vi "Evaluate Alarms.vi"(0 "In Test":bool, 1 "Controller":T2, 2 "Alarm Config":T3, 3 "Data":dbl[](array[numeric]), 4 "Pumps Present":u32, 5 "Trip Counter":i32[](array[numeric]), 6 "Previous Times":u32[](array[numeric]), 7 "Manual CMDs":dbl[](array[numeric]), 9 "Prev ON Times":u32[](array[numeric])) -> (20 "Trip Counter OUT":i32[](array[numeric]), 21 "Previous Times OUT":u32[](array[numeric]), 22 "Alarm Tripped":bool, 23 "Alarm Message":string, 24 "Prev ON Times OUT":u32[](array[numeric]))   [LabVIEW 2019]
uses:
  Controls/Alarm Config.ctl
  Controls/Alarm Definition.ctl
  Controls/Alarm Profile Config.ctl
  Type Defs/Controller Names.ctl
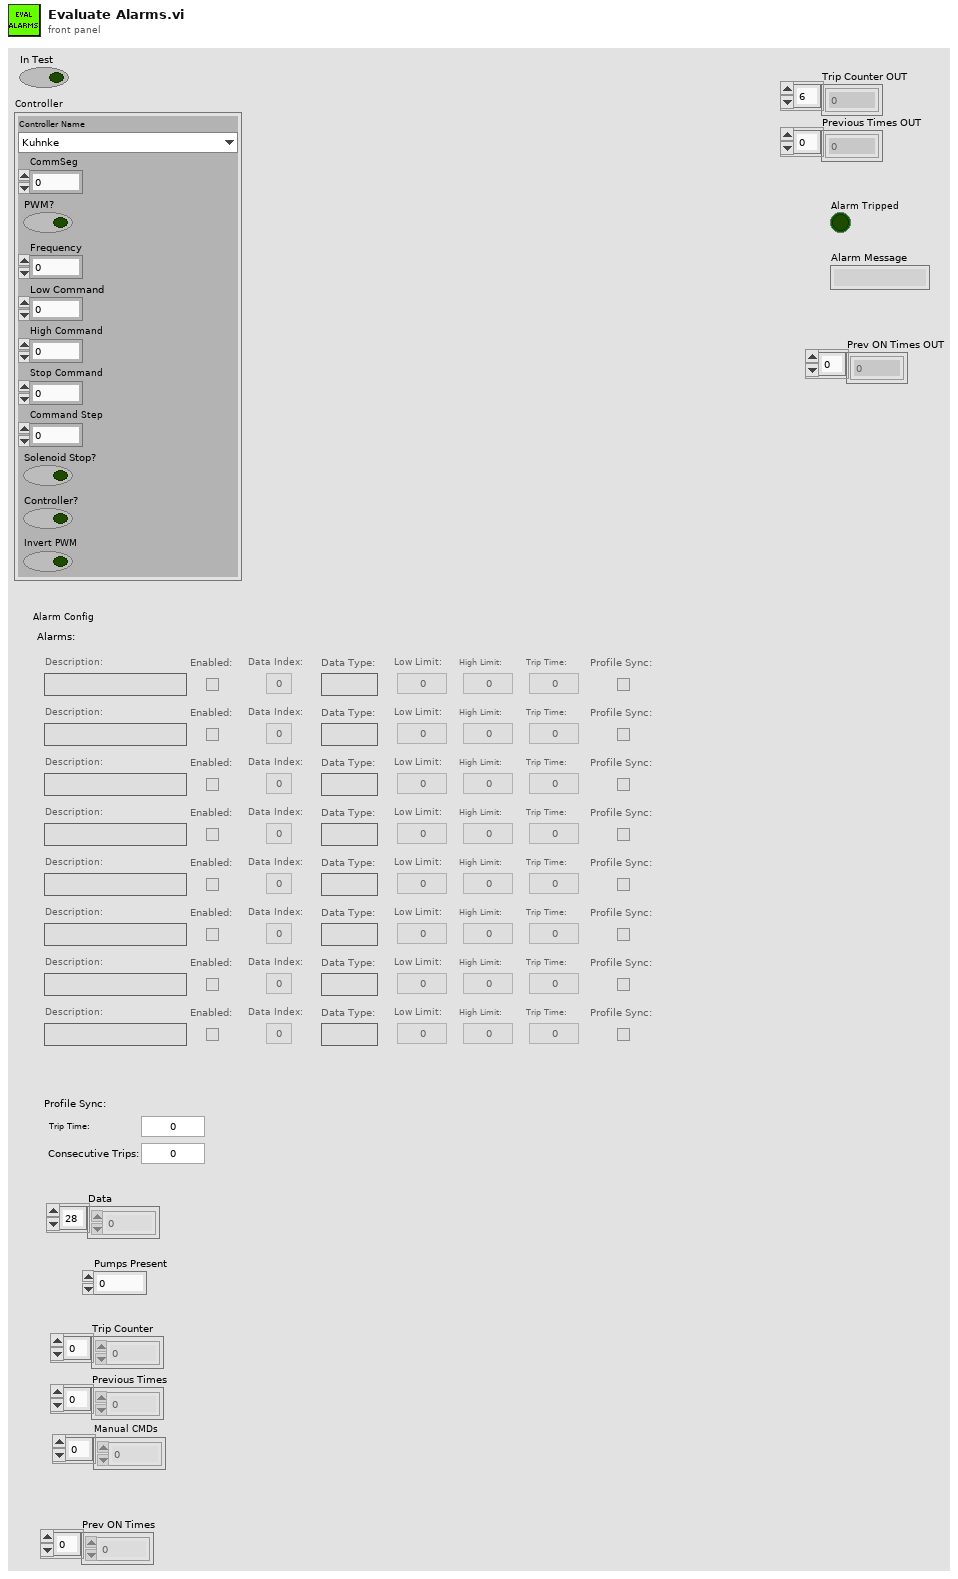
[diagram p1: front panel]
types:
  T1 = typedef "Controller Names.ctl" = enum16{"Kuhnke", "Conti", "Hella BLDC OL PWM", "Hella BLDC Turbine OL PWM", "Helbako", "TI PWM", "PSA", "Hella DC Gas", "Hella DC Diesel", "8 Comm", "10 Comm", "8 Comm Hella", "10 Comm Hella", "8 Comm Omron", "10 Comm Omron", "8 Comm Nissan", "10 Comm Nissan"}
  T2 = cluster{"Controller Name":T1, "CommSeg":i32, "PWM?":bool, "Frequency":i32, "Low Command":dbl, "High Command":dbl, "Stop Command":dbl, "Command Step":dbl, "Solenoid Stop?":bool, "Controller?":bool, "Invert PWM":bool}
  T3 = typedef "Alarm Config.ctl" = cluster{"Alarms:":T4[], "Profile Sync:":T5}
  T4 = typedef "Alarm Definition.ctl" = cluster{"Description:":string, "Enabled:":bool, "Data Index:":i32, "Data Type:":string, "Low Limit:":dbl, "High Limit:":dbl, "Trip Time:":u32, "Profile Sync:":bool}
  T5 = typedef "Alarm Profile Config.ctl" = cluster{"Trip Time:":u32, "Consecutive Trips:":i32}
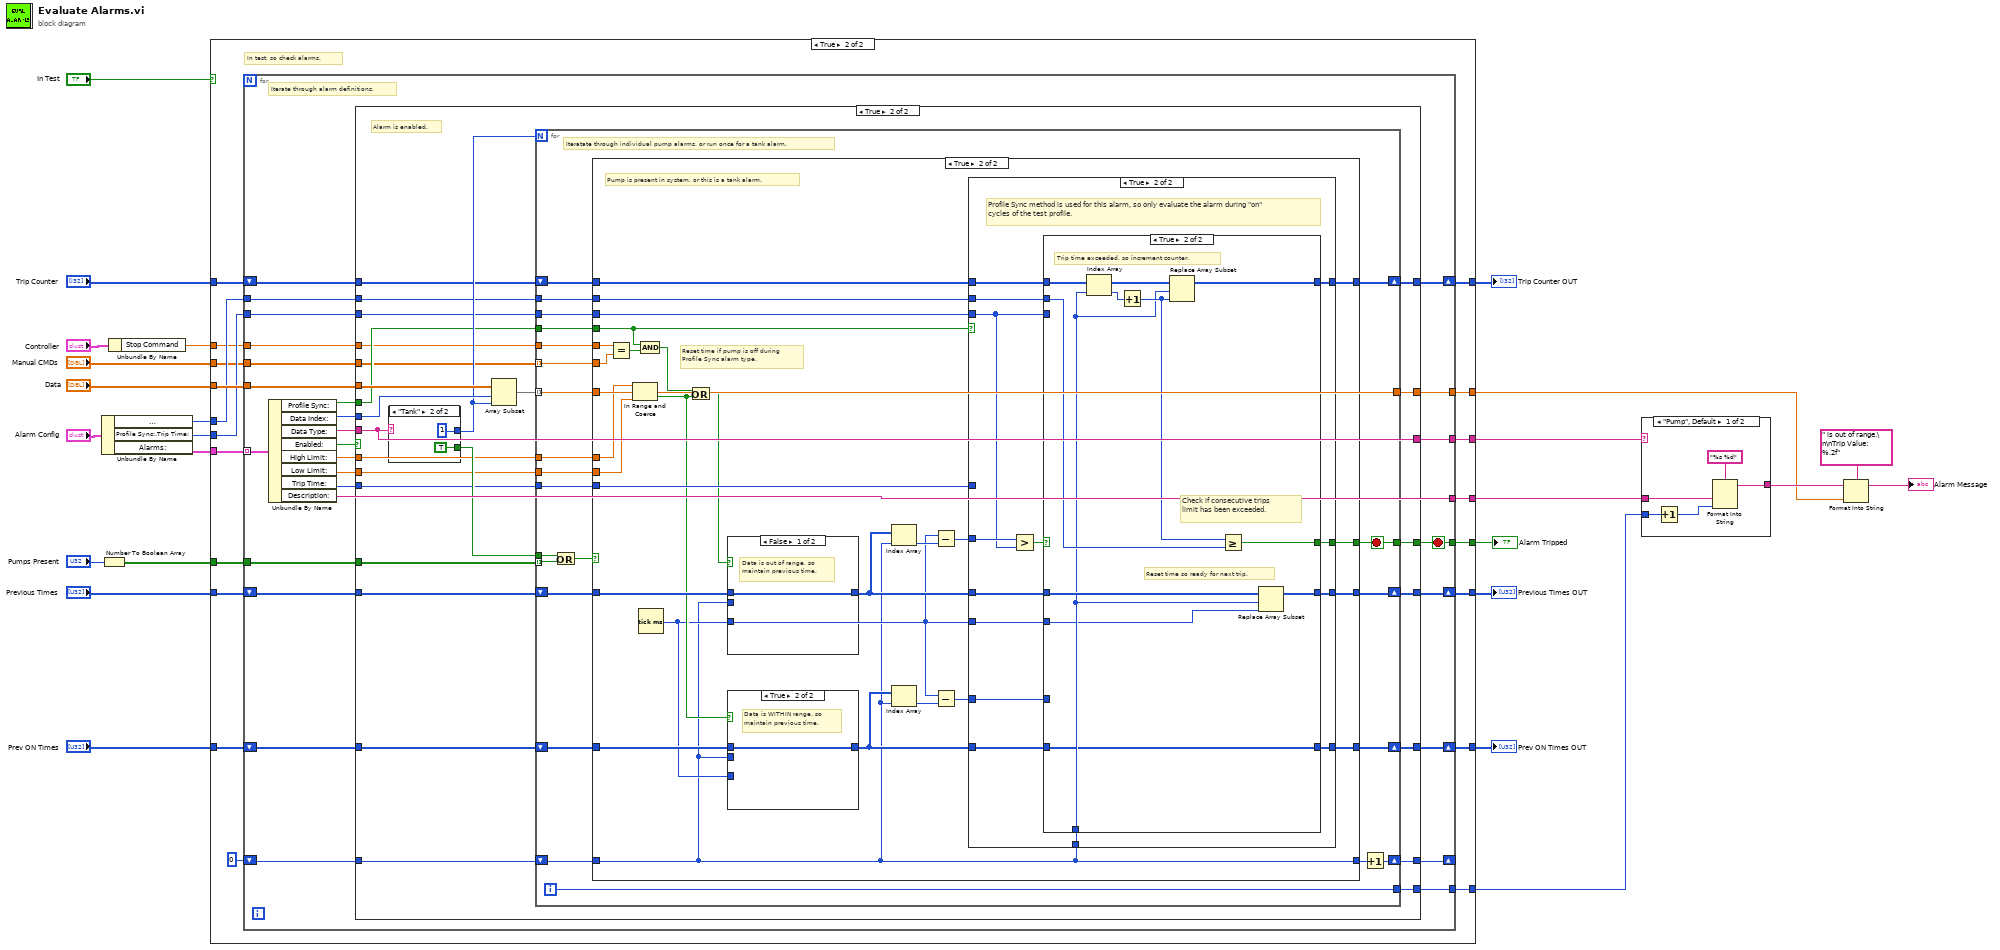
[diagram p0: block diagram]
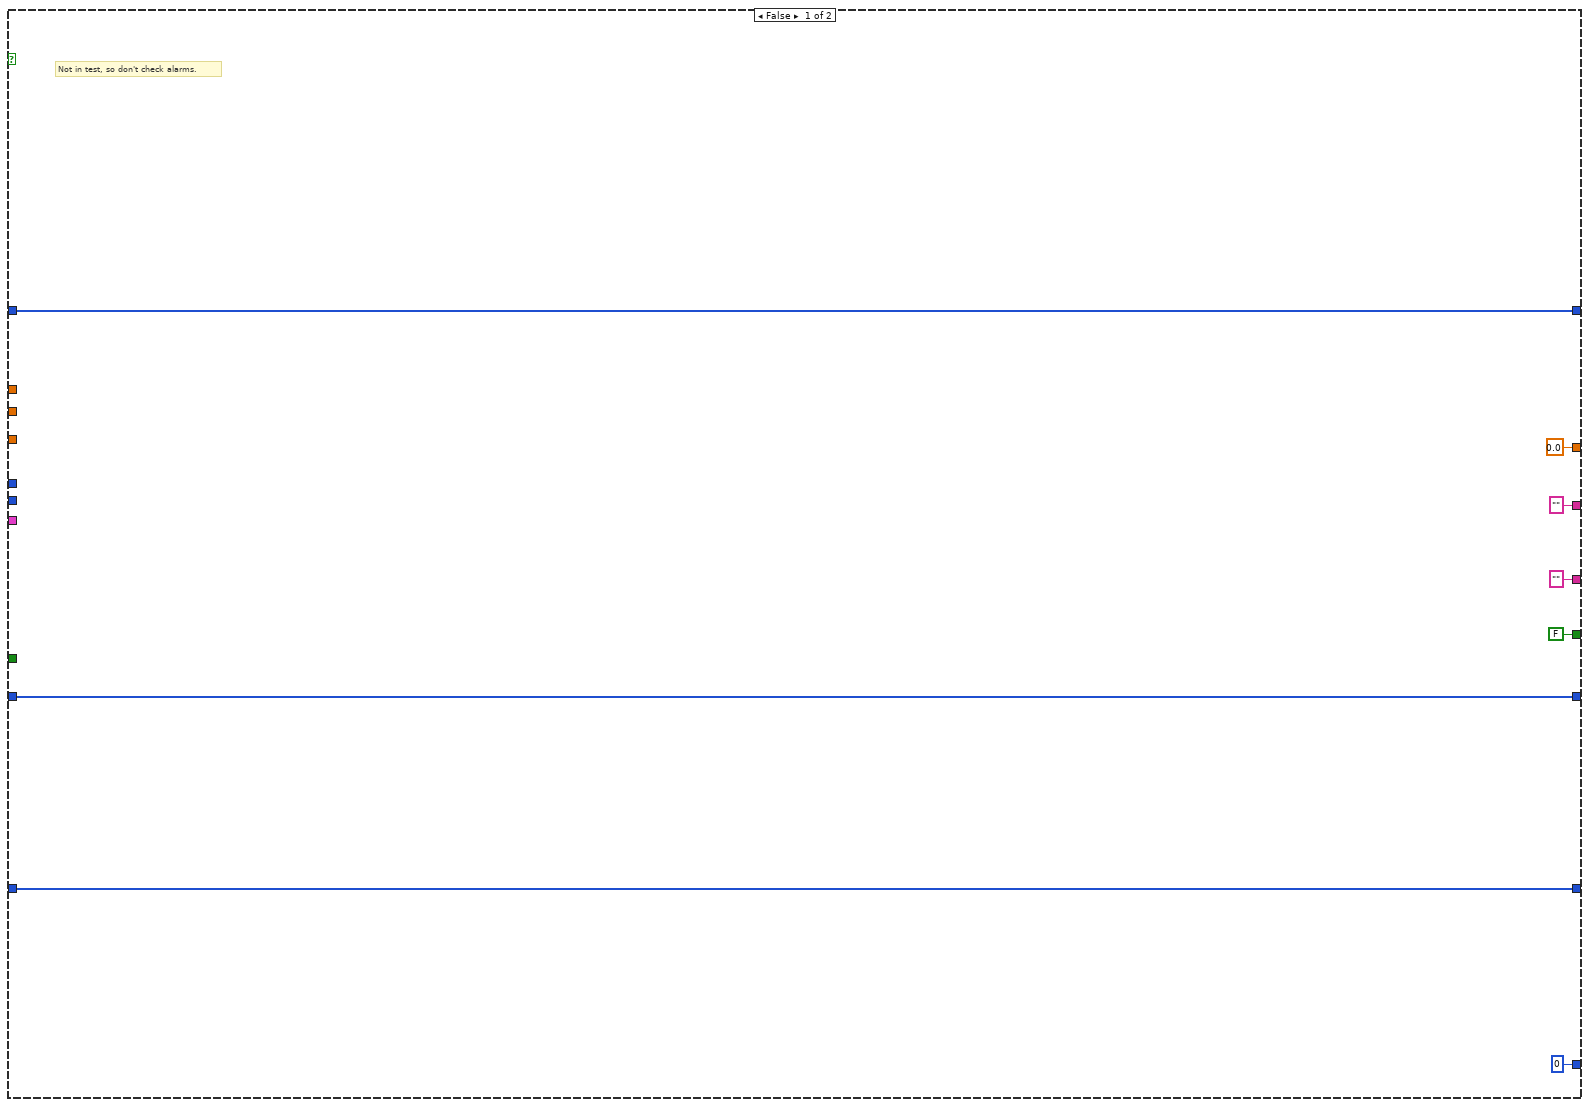
[diagram p3: hidden frame]
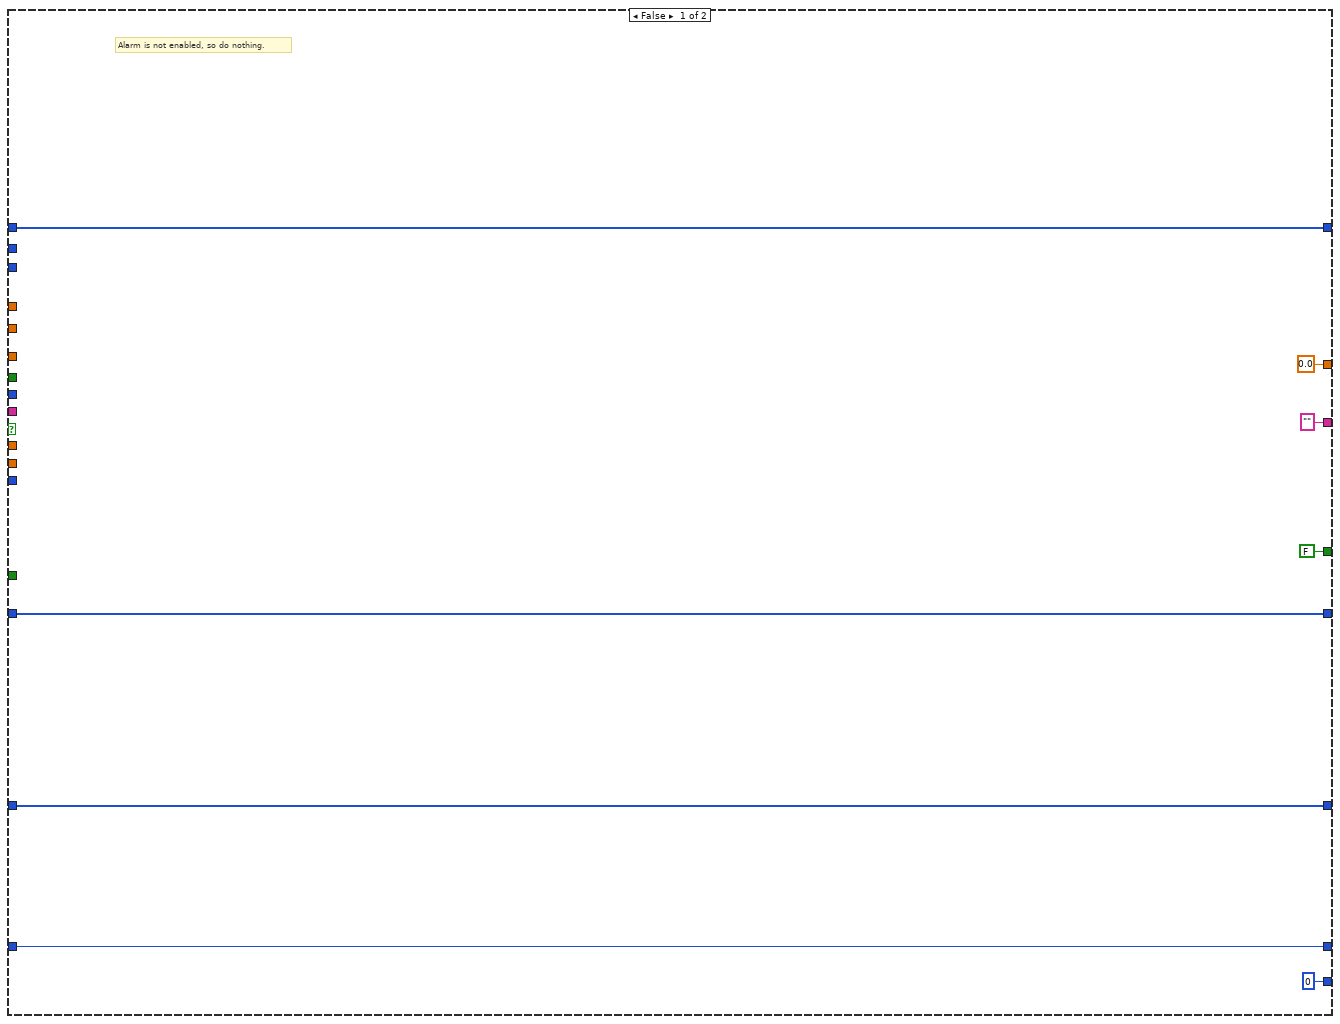
[diagram p4: hidden frame]
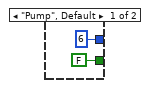
[diagram p5: hidden frame]
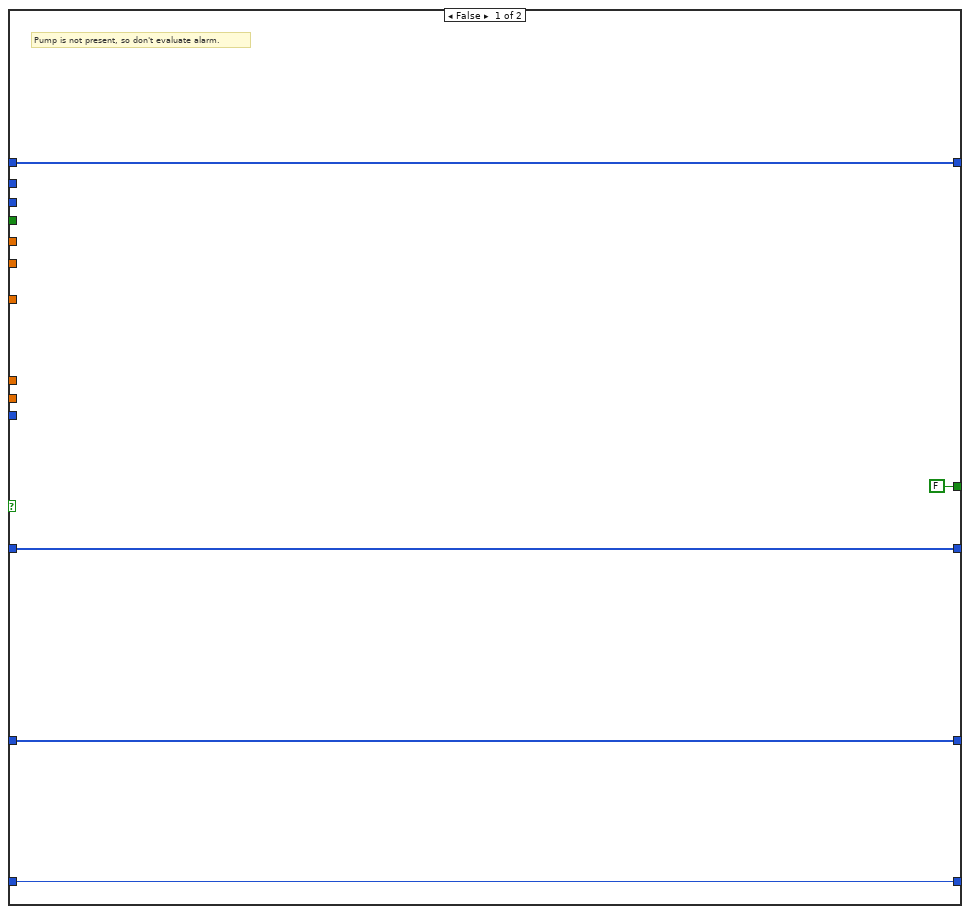
[diagram p6: hidden frame]
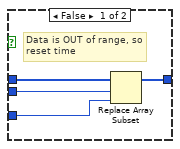
[diagram p7: hidden frame]
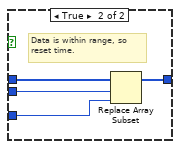
[diagram p8: hidden frame]
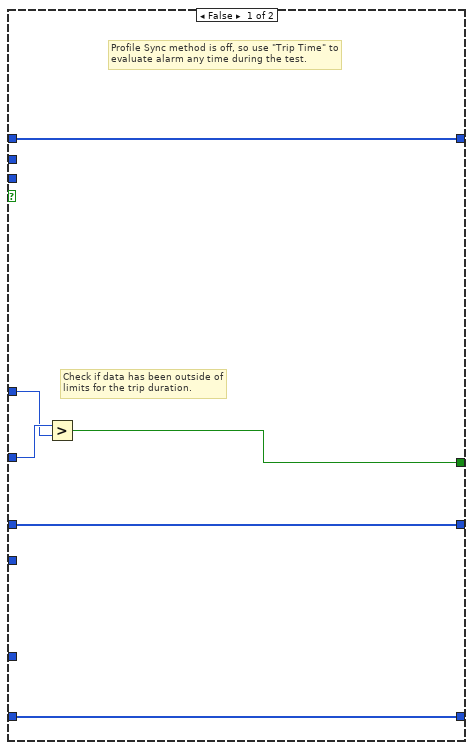
[diagram p9: hidden frame]
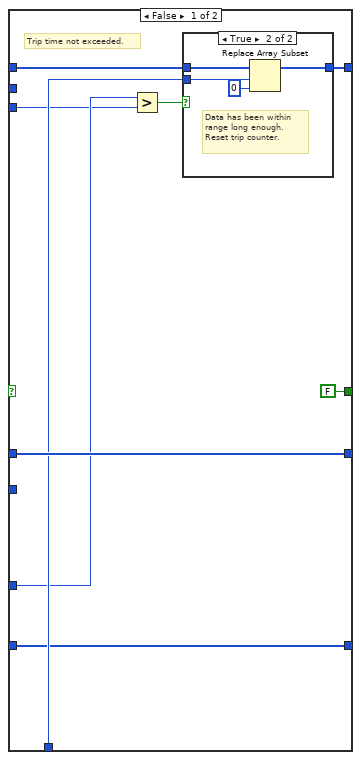
[diagram p10: hidden frame]
diagram:
  n1 = Unbundle By Name("Alarm Config") -> ("Profile Sync:.Consecutive Trips:"=w17:i32, "Profile Sync:.Trip Time:"=w16:u32, "Alarms:"=w22:T4[])
  n2 = Number To Boolean Array(number="Pumps Present") -> (Boolean array=w19:bool[])
  n3 = Unbundle By Name("Controller") -> ("Stop Command"=w15:dbl)
  n4 = case shown="True" "In Test" {
    tunnel: w22 -> [_ w52]
    tunnel: "Data" -> [_ w51]
    tunnel: w19 -> [_ w50]
    tunnel: "Previous Times" -> [w32 w49]
    tunnel: "Trip Counter" -> [w33 w47]
    tunnel: w17 -> [_ w46]
    tunnel: w16 -> [_ w45]
    tunnel: w15 -> [_ w44]
    tunnel: "Manual CMDs" -> [_ w43]
    tunnel: [w33 w42] -> w12
    tunnel: [w32 w41] -> w11
    tunnel: [FALSE w40] -> w10
    tunnel: ["" ("Description:") w39] -> w8
    tunnel: [0 w38] -> w7
    tunnel: ["" ("Data Type:") w37] -> w9
    tunnel: [0.0 w36] -> w4
    tunnel: "Prev ON Times" -> [w26 w35]
    tunnel: [w26 w34] -> w1
    frame False {
      # "Not in test, so don't check alarms."
    }
    frame True {
      # "In test, so check alarms."
      n5 = for {
        tunnel: w52 -> [w79] mode=indexing
        tunnel: w51 -> [w77]
        tunnel: w50 -> [w74]
        shift-right: [w69] -> w41
        shift-left: w49 -> [w70]
        shift-right: [w66] -> _
        shift-left: 0 ("index") -> [w67]
        shift-right: [w64] -> w42
        shift-left: w47 -> [w65]
        tunnel: w46 -> [w63]
        tunnel: w45 -> [w62]
        tunnel: w44 -> [w61]
        tunnel: w43 -> [w60]
        tunnel: [w59] -> w40
        tunnel: [w58] -> w39
        tunnel: [w57] -> w38
        tunnel: [w56] -> w37
        tunnel: [w55] -> w36
        shift-right: [w53] -> w34
        shift-left: w35 -> [w54]
        stop <- w59 stop-if-true
        # "Iterate through alarm definitions."
        n6 = Unbundle By Name(w79) -> ("Profile Sync:"=w68:bool, "Data Index:"=w76:i32, "Data Type:"=w75:string, "Enabled:"=w78:bool, "High Limit:"=w73:dbl, "Low Limit:"=w72:dbl, "Trip Time:"=w71:u32, "Description:"=w58:string)
        n7 = case shown="True" w78 {
          tunnel: w77 -> [_ w113]
          tunnel: w76 -> [_ w112]
          tunnel: w75 -> [_ w91]
          tunnel: w74 -> [_ w109]
          tunnel: w73 -> [_ w108]
          tunnel: w72 -> [_ w107]
          tunnel: w71 -> [_ w106]
          tunnel: w70 -> [w85 w104]
          tunnel: [w85 w103] -> w69
          tunnel: w68 -> [_ w102]
          tunnel: w67 -> [w84 w101]
          tunnel: [w84 w100] -> w66
          tunnel: [FALSE w99] -> w59
          tunnel: w65 -> [w87 w98]
          tunnel: [w87 w97] -> w64
          tunnel: w63 -> [_ w96]
          tunnel: w62 -> [_ w95]
          tunnel: w61 -> [_ w94]
          tunnel: w60 -> [_ w93]
          tunnel: [0 w92] -> w57
          tunnel: ["" ("Data Type:") w91] -> w56
          tunnel: [0.0 w90] -> w55
          tunnel: w54 -> [w80 w89]
          tunnel: [w80 w88] -> w53
          frame False {
            # "Alarm is not enabled, so do nothing."
          }
          frame True {
            # "Alarm is enabled."
            n8 = case shown="\"Tank\"" w91 {
              tunnel: [6 ("length") 1 ("length")] -> w111
              tunnel: [FALSE TRUE] -> w110
              frame "Pump", Default {
              }
              frame "Tank" {
              }
            }
            n9 = Array Subset(array=w113, index=w112, length=w111) -> (w105:dbl[])
            n10 = for {
              N: w111 -> [_]
              tunnel: w110 -> [w140]
              tunnel: w109 -> [w139] mode=indexing
              tunnel: w108 -> [w137]
              tunnel: w107 -> [w136]
              tunnel: w106 -> [w135]
              tunnel: w105 -> [w120] mode=indexing
              shift-right: [w133] -> w103
              shift-left: w104 -> [w134]
              tunnel: w102 -> [w132]
              shift-right: [w122] -> w100
              shift-left: w101 -> [w131]
              tunnel: [w130] -> w99
              shift-right: [w128] -> w97
              shift-left: w98 -> [w129]
              tunnel: w96 -> [w127]
              tunnel: w95 -> [w126]
              tunnel: w94 -> [w125]
              tunnel: w93 -> [w124] mode=indexing
              tunnel: [w121] -> w92
              tunnel: [w120] -> w90
              shift-right: [w118] -> w88
              shift-left: w89 -> [w119]
              i -> [w121]
              stop <- w130 stop-if-true
              # "Iteratate through individual pump alarms, or run once for a tank alarm."
              n11 = Or(x=w140, y=w139) -> (x .or. y?=w138:bool)
              n12 = case shown="True" w138 {
                tunnel: w137 -> [_ w172]
                tunnel: w136 -> [_ w171]
                tunnel: w135 -> [_ w166]
                tunnel: w120 -> [_ w173]
                tunnel: w134 -> [w143 w170]
                tunnel: [w143 w154] -> w133
                tunnel: w132 -> [_ w158]
                tunnel: w131 -> [w142 w146]
                tunnel: [w142 w146] -> w123
                tunnel: [FALSE w168] -> w130
                tunnel: w129 -> [w145 w165]
                tunnel: [w145 w164] -> w128
                tunnel: w127 -> [_ w163]
                tunnel: w126 -> [_ w162]
                tunnel: w125 -> [_ w161]
                tunnel: w124 -> [_ w160]
                tunnel: w119 -> [w141 w152]
                tunnel: [w141 w149] -> w118
                frame False {
                  # "Pump is not present, so don't evaluate alarm."
                }
                frame True {
                  # "Reset time if pump is off during\nProfile Sync alarm type."
                  # "Pump is present in system, or this is a tank alarm."
                  n13 = Equal?(x=w161, y=w160) -> (x = y?=w159:bool)
                  n14 = In Range and Coerce(upper limit=w172, x=w173, lower limit=w171) -> (In Range?=w153:bool)  [unwired: 1 out]
                  n15 = And(x=w158, y=w159) -> (x .and. y?=w157:bool)
                  n16 = Tick Count (ms)() -> (millisecond timer value=w150:u32)
                  n17 = Or(x=w157, y=w153) -> (x .or. y?=w156:bool)
                  n18 = case shown="False" w156 {
                    tunnel: w170 -> [w179 w183]
                    tunnel: [w179 w182] -> w155
                    tunnel: w146 -> [_ w181]
                    tunnel: w150 -> [_ w180]
                    frame False {
                      # "Data is out of range, so\nmaintain previous time."
                    }
                    frame True {
                      # "Data is within range, so\nreset time."
                      n19 = Replace Array Subset(array=w183, new element=w180, index=w181) -> (w182:u32[])
                    }
                  }
                  n20 = case shown="True" w153 {
                    tunnel: w152 -> [w177 w178]
                    tunnel: [w176 w178] -> w148
                    tunnel: w146 -> [w175 _]
                    tunnel: w150 -> [w174 _]
                    frame False {
                      # "Data is OUT of range, so\nreset time"
                      n21 = Replace Array Subset(array=w177, new element=w174, index=w175) -> (w176:u32[])
                    }
                    frame True {
                      # "Data is WITHIN range, so\nmaintain previous time."
                    }
                  }
                  n22 = Index Array(array=w155, index=w146) -> (element=w169:u32)
                  n23 = Index Array(array=w148, index=w146) -> (element=w151:u32)
                  n24 = Subtract(x=w150, y=w169) -> (x-y=w167:u32)
                  n25 = Subtract(x=w150, y=w151) -> (x-y=w147:u32)
                  n26 = case shown="True" w158 {
                    tunnel: [w187 w197] -> w168
                    tunnel: w167 -> [w189 w203]
                    tunnel: w166 -> [w188 _]
                    tunnel: w165 -> [w186 w202]
                    tunnel: [w186 w201] -> w164
                    tunnel: w163 -> [_ w198]
                    tunnel: w162 -> [_ w190]
                    tunnel: w146 -> [_ w199]
                    tunnel: w155 -> [w185 w196]
                    tunnel: [w185 w195] -> w154
                    tunnel: w150 -> [_ w194]
                    tunnel: w148 -> [w184 w193]
                    tunnel: [w184 w192] -> w149
                    tunnel: w147 -> [_ w191]
                    frame False {
                      # "Check if data has been outside of\nlimits for the trip duration."
                      # "Profile Sync method is off, so use \"Trip Time\" to\nevaluate alarm any time during the test."
                      n27 = Greater?(x=w189, y=w188) -> (0:w187:bool)
                    }
                    frame True {
                      # "Profile Sync method is used for this alarm, so only evaluate the alarm during \"on\" cycles of the test profile."
                      n28 = Greater?(x=w203, y=w190) -> (0:w200:bool)
                      n29 = case shown="True" w200 {
                        tunnel: [w209 w228] -> w201
                        tunnel: w202 -> [w210 w227]
                        tunnel: w199 -> [w208 w220]
                        tunnel: w198 -> [_ w224]
                        tunnel: [FALSE w223] -> w197
                        tunnel: w196 -> [w211 w222]
                        tunnel: [w211 w221] -> w195
                        tunnel: w194 -> [_ w219]
                        tunnel: [w204 w218] -> w192
                        tunnel: w193 -> [w204 w218]
                        tunnel: w191 -> [w207 _]
                        tunnel: w190 -> [w206 _]
                        frame False {
                          # "Trip time not exceeded."
                          n30 = Greater?(x=w207, y=w206) -> (0:w205:bool)
                          n31 = case shown="True" w205 {
                            tunnel: w210 -> [w213 w217]
                            tunnel: [w213 w216] -> w209
                            tunnel: w208 -> [_ w215]
                            frame False {
                              # "Data has NOT come\ncome back into range\nlong enough.\nMaintain counters."
                            }
                            frame True {
                              # "Data has been within\nrange long enough. \nReset trip counter."
                              n32 = Replace Array Subset(array=w217, new element=0 ("new element/subarray"), index=w215) -> (w216:i32[])
                            }
                          }
                        }
                        frame True {
                          # "Reset time so ready for next trip."
                          # "Check if consecutive trips limit has been exceeded."
                          # "Trip time exceeded, so increment counter."
                          n33 = Index Array(array=w227, index=w220) -> (element=w226:i32)
                          n34 = Increment(x=w226) -> (x+1=w225:i32)
                          n35 = Replace Array Subset(array=w227, new element=w225, index=w220) -> (w228:i32[])
                          n36 = Greater Or Equal?(x=w225, y=w224) -> (x >= y?=w223:bool)
                          n37 = Replace Array Subset(array=w222, new element=w219, index=w220) -> (w221:u32[])
                        }
                      }
                    }
                  }
                }
              }
              n38 = Increment(x=w123) -> (x+1=w122:i32)
            }
          }
        }
      }
    }
  }
  "Trip Counter OUT" <- w12
  "Previous Times OUT" <- w11
  "Alarm Tripped" <- w10
  "Prev ON Times OUT" <- w1
  n39 = case shown="\"Pump\", Default" w9 {
    tunnel: w8 -> [w231 w234]
    tunnel: w7 -> [w230 _]
    tunnel: [w232 w234] -> w5
    frame "Pump", Default {
      n40 = Increment(x=w230) -> (x+1=w229:i32)
      n41 = Format Into String(format string="%s %d", w231, w229) -> (resulting string=w232:string)  [unwired: 2 in, 1 out]
    }
    frame "Tank" {
    }
  }
  n42 = Format Into String(format string=" is out of range.\n\nTrip Value:  %.2f", initial string=w5, w4) -> (resulting string=→"Alarm Message":string)  [unwired: 1 in, 1 out]
